vi "Get Scope Errors.vi"(7 "scope":T2, 8 "error in (no error)":errorcluster, 11 "error list <top> in":variant) -> (0 "error out":errorcluster, 1 "attributes":string[](array[string]), 2 "errors":T1[](array[typedef]), 3 "error list <top> out":variant, 4 "error codes":i32[](array[numeric]))   [LabVIEW 2017]
uses:
  Scope.ctl
  Error File Management/Controls/NI Error.ctl
  Error File Management/Error File Management.lvlib
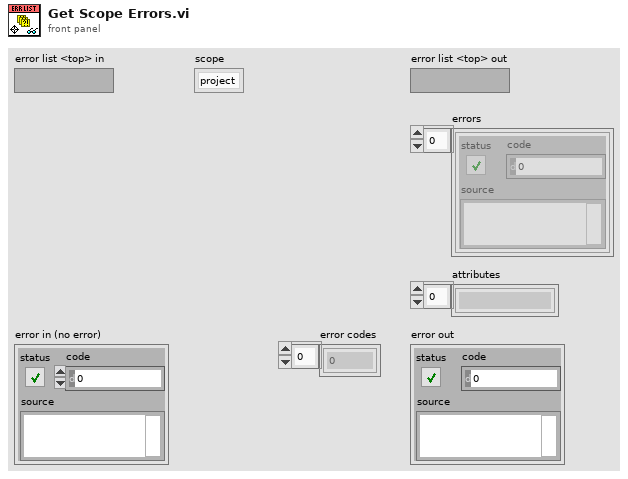
[diagram p1: front panel]
types:
  T1 = typedef "Error File Management.lvlib/NI Error.ctl" = errorcluster
  T2 = typedef "Scope.ctl" = enum16{"project", "global"}
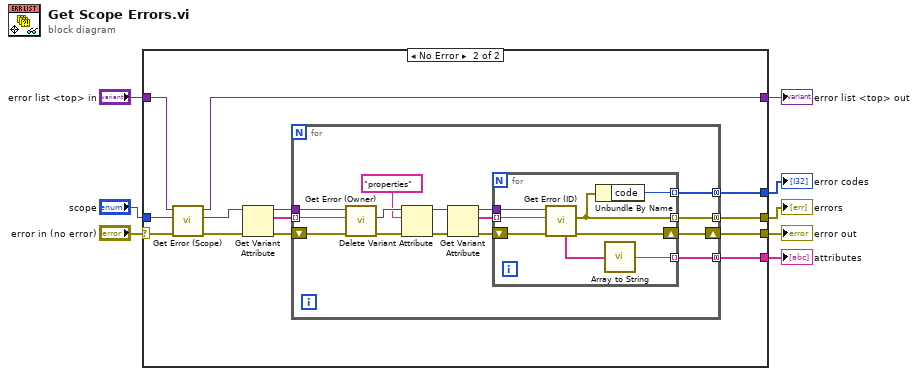
[diagram p0: block diagram]
diagram:
  n1 = case shown="No Error" "error in (no error)" {
    selector: "error in (no error)" -> [w10 w16]
    tunnel: "scope" -> [_ w23]
    tunnel: [w10 w17] -> w6
    tunnel: "error list <top> in" -> [w9 w15]
    tunnel: [w9 w14] -> w4
    tunnel: [_ w13] -> w3
    tunnel: [_ w12] -> w2
    tunnel: [_ w11] -> w1
    frame Error {
    }
    frame No Error {
      n2 = call "Get Error (Scope).vi"("error in (no error)"=w16, "scope"=w23, "error list <top>"=w15) -> ("error out"=w18:errorcluster, "error list <scope>"=w20:variant, "error list <top> dup"=w14:variant)  [unwired: 5 in, 1 out]
      n3 = Get Variant Attribute(Variant=w20, error in=w18) -> (duplicate Variant=w21:variant, names=w22:string[], error out=w19:errorcluster)  [unwired: 2 in, 1 out]
      n4 = for {
        shift-right: [w35] -> w17
        shift-left: w19 -> [w38]
        tunnel: w22 -> [w34] mode=indexing
        tunnel: w21 -> [w37]
        tunnel: [w28] -> w12 mode=concatenating
        tunnel: [w27] -> w13 mode=concatenating
        tunnel: [w26] -> w11 mode=concatenating
        n5 = call "Get Error (Owner).vi"("error in (no error)"=w38, "owner"=w34, "error list <scope>"=w37) -> ("error out"=w36:errorcluster, "error list <owner>"=w25:variant)  [unwired: 5 in, 2 out]
        n6 = Delete Variant Attribute(4:w36, 6:"properties" ("name"), 7:w25) -> (0:w30:errorcluster, 3:w29:variant)  [unwired: 1 out]
        n7 = Get Variant Attribute(Variant=w29, error in=w30) -> (duplicate Variant=w32:variant, names=w31:string[], error out=w33:errorcluster)  [unwired: 2 in, 1 out]
        n8 = for {
          shift-right: [w45] -> w35
          shift-left: w33 -> [w46]
          tunnel: w31 -> [w43] mode=indexing
          tunnel: [w42] -> w28 mode=indexing
          tunnel: w32 -> [w44]
          tunnel: [w41] -> w27 mode=indexing
          tunnel: [w40] -> w26 mode=indexing
          n9 = call "Get Error (ID).vi"("error in (no error)"=w46, "ID"=w43, "error list <owner>"=w44) -> ("error out"=w45:errorcluster, "error"=w42:T1, "attributes"=w39:string[])  [unwired: 4 in, 2 out]
          n10 = Unbundle By Name(w42) -> ("code"=w41:i32)
          n11 = call "Array to String.vi"("array"=w39) -> ("string"=w40:string)  [unwired: 1 in]
        }
      }
    }
  }
  "error out" <- w6
  "error list <top> out" <- w4
  "errors" <- w2
  "error codes" <- w3
  "attributes" <- w1
